vi "Fire User Event.vi"(8 "error in (no error)":errorcluster caption="에러 입력(에러 없음)", 11 "User Event":refnum<user-event>) -> (0 "error out":errorcluster caption="에러 출력")   [LabVIEW 2018, in "User Event.lvlib"]
doc: "정지 이벤트를 보내서 이벤트 핸들링 루프를 정지합니다."
uses:
  User Event.lvlib
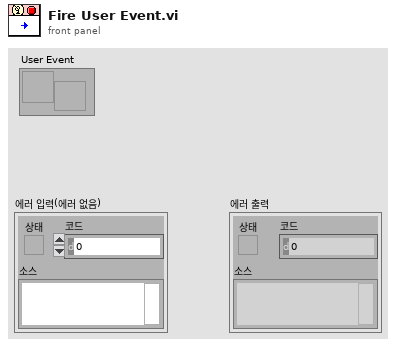
[diagram p1: front panel]
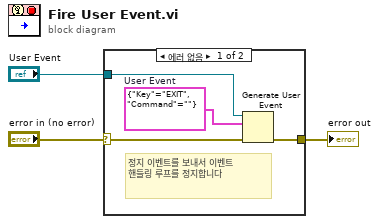
[diagram p0: block diagram]
diagram:
  n1 = case shown="에러 없음" "error in (no error)" {
    selector: "error in (no error)" -> [w5 w8]
    tunnel: [w7 w8] -> w3
    tunnel: "User Event" -> [w6 _]
    frame No Error {
      w4 = cluster{"Key":string, "Command":string} {"Key"="EXIT", "Command"=""}  # User Event
      # "정지 이벤트를 보내서 이벤트 핸들링 루프를 정지합니다"
      n2 = Generate User Event(user event=w6, event data cluster=w4, error in=w5) -> (error out=w7:errorcluster)  [unwired: 1 in, 1 out]
    }
    frame Error {
    }
  }
  "error out" <- w3
